vi "Waveform Settings Read.vi"(4 "error in (no error)":errorcluster, 6 "Container State":T2, 7 "Display State In":T1) -> (0 "error out":errorcluster, 2 "Value":T3={"Type"=enum."Sine", "Periods"=0.0, "Points"=0, "Offset"=0.0, "Amplitdue"=0.0, "Starting Phase"=0.0, "func"=""}, 3 "Display State Out":T1)   [LabVIEW 2012, in "Waveform Control.xctl"]
uses:
  Waveform Control.xctl
  <vilib>/_xctls/Container State.ctl
  subvis/FP Controls.ctl
  subvis/Function Types.ctl
  Controls/State.ctl
  Controls/Volatile State Ops.ctl
  <vilib>/_xctls/XControlSupport.lvlib
panel:
  # "Replace the Value Indicator below with an Indicator of desired type.\nDo not remove this Indicator or the others from the connector pane. \nDo not change the connector pane pattern.\nThe Value Indicator should always be the second terminal from top on the output side in the connector pane."
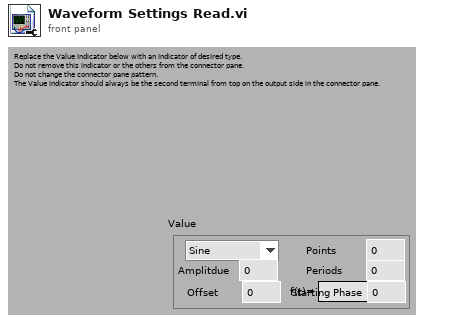
[diagram p1: front panel]
types:
  T1 = typedef "Waveform Control.xctl/State.ctl" = cluster{"Name":string}
  T2 = typedef "XControlSupport.lvlib/Container State.ctl" = cluster{"Indicator?":bool, "Run Mode?":bool, " Refnum":refnum<vi>}
  T3 = typedef "Waveform Control.xctl/FP Controls.ctl" = cluster{"Type":T4, "Periods":dbl, "Points":i32, "Offset":dbl, "Amplitdue":dbl, "Starting Phase":dbl, "func":string}
  T4 = typedef "Waveform Control.xctl/Function Types.ctl" = enum16{"Level", "Sine", "Triangle", "Ramp", "Saw Tooth", "Square", "Function"}
  T5 = typedef "Waveform Control.xctl/Volatile State Ops.ctl" = enum16{"Read", "Write", "Update State from Data"}
  T6 = typedef "Waveform Control.xctl/Waveform State.ctl" = cluster{"Show Axes":bool, "Show Y=0":bool, "Controls":T3, "Show Current Location":bool, "Current Location":i32, "dt":dbl, "t0":timestamp, "Amplitude Format String":string}
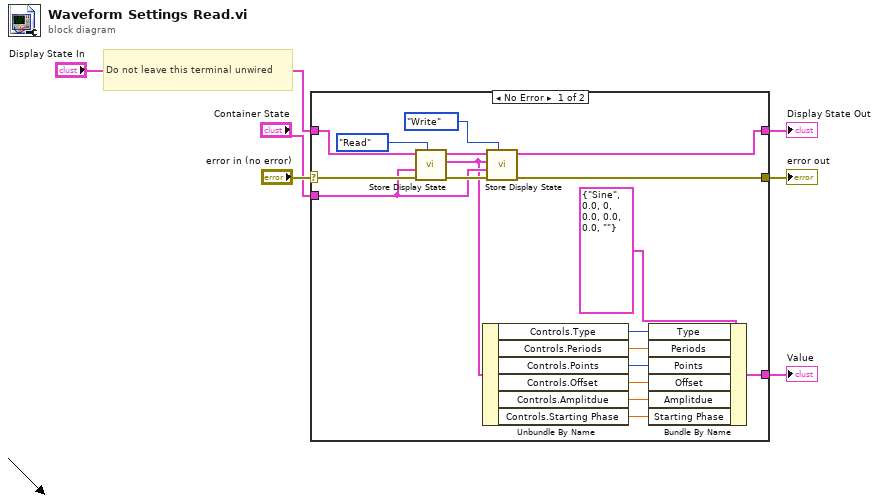
[diagram p0: block diagram]
diagram:
  # "Do not leave this terminal unwired"
  n1 = case shown="No Error" "error in (no error)" {
    selector: "error in (no error)" -> [w22 w26]
    tunnel: "Display State In" -> [w24 w25]
    tunnel: [w21 w26] -> w4
    tunnel: [w18 w25] -> w2
    tunnel: [w10 _] -> w3
    tunnel: "Container State" -> [w9 _]
    frame No Error {
      n2 = call "Store Display State.vi"("Operation In"=Volatile_State_Ops."Read" ("Operation"), "Error In (no Error) In"=w22, "Container State In"=w9, "State In"=w24) -> ("Error Out"=w23:errorcluster, "Waveform State Out"=w7:T6, "Display State Out"=w8:T1)  [unwired: 2 in, 3 out]
      n3 = Unbundle By Name(w7) -> ("Controls.Type"=w17:T4, "Controls.Periods"=w16:dbl, "Controls.Points"=w15:i32, "Controls.Offset"=w14:dbl, "Controls.Amplitdue"=w13:dbl, "Controls.Starting Phase"=w12:dbl)
      n4 = call "Store Display State.vi"("Operation In"=Volatile_State_Ops."Write" ("Operation"), "Error In (no Error) In"=w23, "Container State In"=w9, "Waveform State In"=w7, "State In"=w8) -> ("Error Out"=w21:errorcluster, "Display State Out"=w18:T1)  [unwired: 1 in, 4 out]
      n5 = Bundle By Name(cluster=T3 {"Type"=enum."Sine", "Periods"=0.0, "Points"=0, "Offset"=0.0, "Amplitdue"=0.0, "Starting Phase"=0.0, "func"=""} ("Controls"), "Type"=w17, "Periods"=w16, "Points"=w15, "Offset"=w14, "Amplitdue"=w13, "Starting Phase"=w12) -> (w10:T3)
    }
    frame Error {
    }
  }
  "error out" <- w4
  "Value" <- w3
  "Display State Out" <- w2
